vi "STM Read Meta Data.vi"   [LabVIEW 2015, in "J1939 Addon Shared.lvlib"]
doc: "This VI reads the meta data information from a remote computer. Use this VI to retrieve the variable names and types that a remote computer exports.\n\nThis VI parses the data and returns a cluster containing the meta data information."
uses:
  J1939 Addon Shared.lvlib
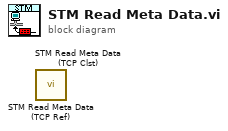
[diagram p0: block diagram]
diagram:
  n1 = call "STM Read Meta Data (TCP Ref).vi"() -> ()  [unwired: 9 in, 3 out]
  n2 = call "STM Read Meta Data (TCP Clst).vi"() -> ()  [unwired: 9 in, 3 out]
